vi "Write tipo_generador.vi"(8 "error in (no error)":errorcluster, 10 "tipo_generador":string, 11 "Prueba in":refnum<class "Prueba.lvclass">) -> (0 "error out":errorcluster, 3 "Prueba out":refnum<class "Prueba.lvclass">)   [LabVIEW 2019, in "Prueba.lvclass"]
uses:
  Prueba.lvclass
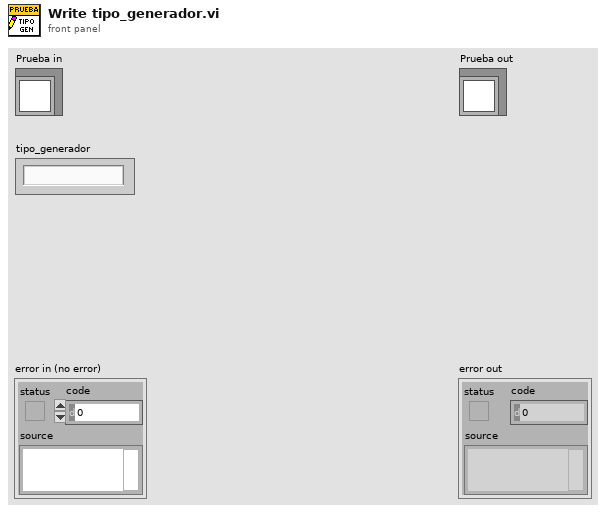
[diagram p1: front panel]
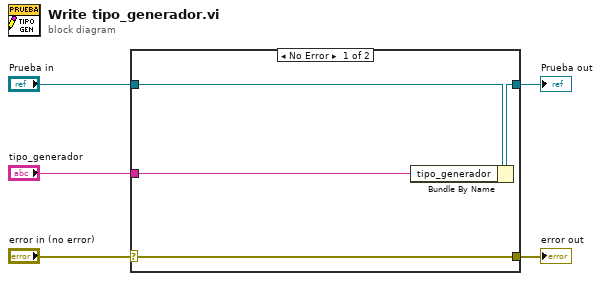
[diagram p0: block diagram]
diagram:
  n1 = case shown="No Error" "error in (no error)" {
    selector: "error in (no error)" -> [w9 w10]
    tunnel: [w9 w10] -> w4
    tunnel: [w7 w11] -> w2
    tunnel: "Prueba in" -> [w8 w11]
    tunnel: "tipo_generador" -> [w6 _]
    frame No Error {
      n2 = Bundle By Name(cluster=w8, "tipo_generador"=w6) -> (w7:refnum<class "Prueba.lvclass">)
    }
    frame Error {
    }
  }
  "error out" <- w4
  "Prueba out" <- w2
